vi "1D array_square.vi"(8 "error in (no error)":errorcluster caption="错误输入（无错误）", 9 "array2":dbl[](array[numeric]), 10 "array1":dbl[](array[numeric])) -> (0 "error out":errorcluster caption="错误输出", 2 "dis2":dbl)   [LabVIEW 2013]
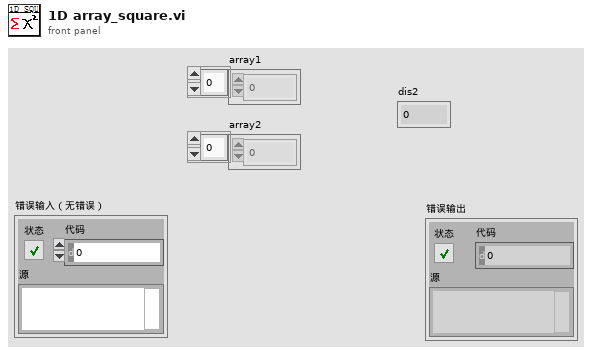
[diagram p1: front panel]
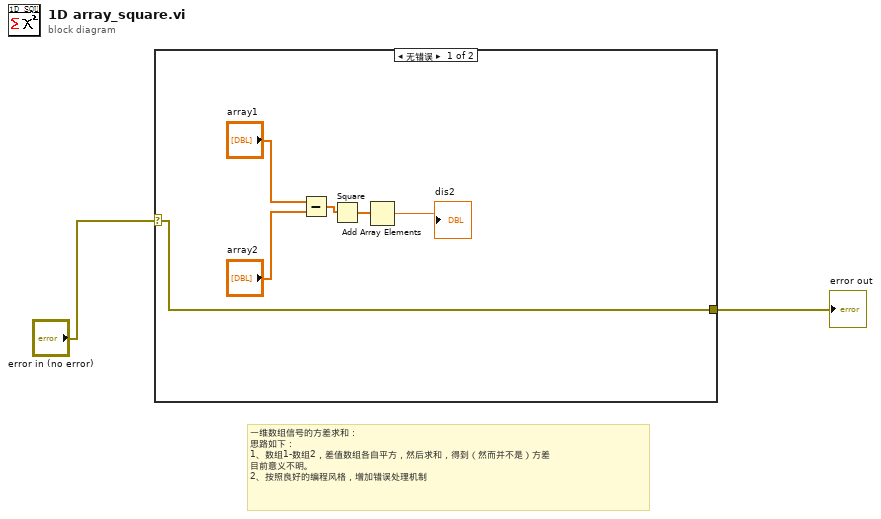
[diagram p0: block diagram]
diagram:
  # "一维数组信号的方差求和：\n思路如下：\n1、数组1-数组2，差值数组各自平方，然后求和，得到（然而并不是）方差\n目前意义不明。\n2、按照良好的编程风格，增加错误处理机制"
  n1 = case shown="无错误" "error in (no error)" {
    selector: "error in (no error)" -> [w3 w9]
    tunnel: [w3 w9] -> w1
    frame No Error {
      n2 = Subtract(x="array1", y="array2") -> (x-y=w6:dbl[])
      n3 = Square(x=w6) -> (x^2=w7:dbl[])
      n4 = Add Array Elements(numeric array=w7) -> (sum=→"dis2":dbl)
    }
    frame Error {
    }
  }
  "error out" <- w1
